vi "Tektronix AFG 3000 Series Generate Arbitrary Waveform Pulse.vi"() -> ()   [LabVIEW 2019]
doc: "Demonstrates how to configure then create an arbitrary waveform."
uses:
  <userlib>/Tektronix AFG 3000 Series/Tektronix AFG 3000 Series.lvlib
panel:
  out "Delta(ms)":u32
  out "taille(s)":i32
  out "periode(us)":dbl
  in  "LowLevel(V)":dbl
  in  "HighLevel(V)":dbl=1.0
  in  "Rise time(us)":dbl=1.0
  in  "Tau2 lenght(us)":dbl=1.0
  in  "Tau1 lenght(us)":dbl=1.0
  in  "Middle pulse lenght(us)":dbl=1.0
  in  "Init pulse lenght(us)":dbl=1.0
  out "Arbitrary Waveform Data":dbl[](array[numeric])
  out "Frequency (1000 Hz)":dbl=1000.0
  in  "DC Offset (0 V)":dbl
  in  "Gain (1 V)":dbl=1.0
  in  "Arbitrary Waveform Name (0: USER1)":u16(ring) items=["USER1", "USER2", "USER3", "USER4"]
  in  "Channel (0: Channel 1)":u16(ring) items=["Channel 1", "Channel 2"]
  in  "VISA resource name":refnum<visa-resource-name>
  # "(c) 2006-2012 National Instruments.  ALL RIGHTS RESERVED."
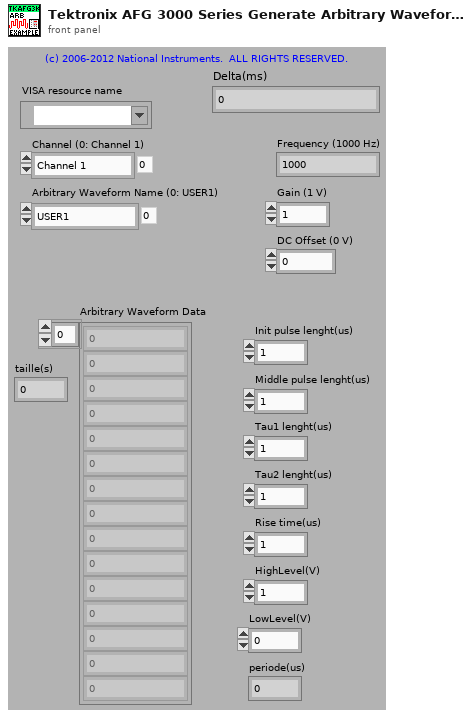
[diagram p1: front panel]
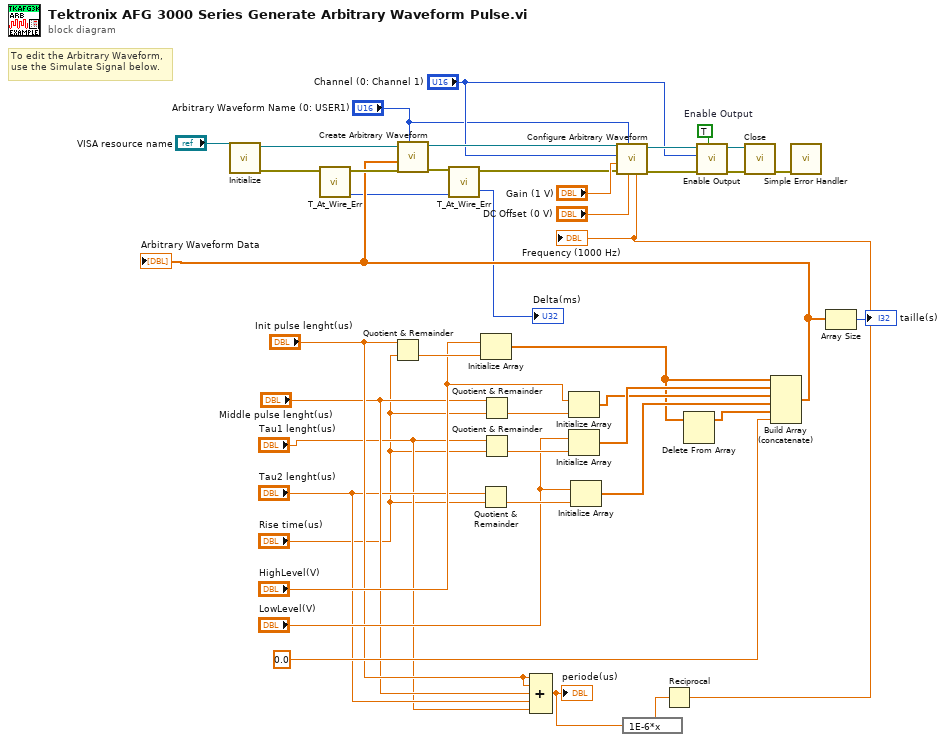
[diagram p0: block diagram]
diagram:
  w35 = TRUE  # Enable Output
  # "To edit the Arbitrary Waveform, use the Simulate Signal below."
  n1 = call <userlib>:"Initialize.vi"("VISA resource name"="VISA resource name") -> ("error out"=w9:errorcluster, "VISA resource name out"=w34:refnum<visa-resource-name>)  [unwired: 9 in]
  n2 = call <userlib>:"T_At_Wire_Err.vi"("error in (no error)"=w9) -> ("Clock(ms)"=w2:u32, "error out"=w8:errorcluster)  [unwired: 8 in, 1 out]
  n3 = Quotient & Remainder(x="Init pulse lenght(us)", y="Rise time(us)") -> (floor(x/y)=w29:dbl)  [unwired: 1 out]
  n4 = Initialize Array("HighLevel(V)", w29) -> (w16:dbl[])
  n5 = Quotient & Remainder(x="Tau2 lenght(us)", y="Rise time(us)") -> (floor(x/y)=w25:dbl)  [unwired: 1 out]
  n6 = Quotient & Remainder(x="Middle pulse lenght(us)", y="Rise time(us)") -> (floor(x/y)=w28:dbl)  [unwired: 1 out]
  n7 = Quotient & Remainder(x="Tau1 lenght(us)", y="Rise time(us)") -> (floor(x/y)=w26:dbl)  [unwired: 1 out]
  n8 = Compound Arithmetic op=ADD("Init pulse lenght(us)", "Init pulse lenght(us)", "Middle pulse lenght(us)", "Tau2 lenght(us)", "Tau1 lenght(us)") -> (w13:dbl)
  "periode(us)" <- w13
  n9 = Initialize Array("HighLevel(V)", w28) -> (w22:dbl[])
  n10 = Initialize Array("LowLevel(V)", w26) -> (w23:dbl[])
  n11 = Initialize Array("LowLevel(V)", w25) -> (w21:dbl[])
  n12 = expression code="1E-6*x"(w13) -> (w10:dbl)
  n13 = Reciprocal(x=w10) -> (1/x=w12:dbl)
  "Frequency (1000 Hz)" <- w12
  n14 = Delete From Array(array=w16) -> (array with subset deleted=w15:dbl[])  [unwired: 2 in, 1 out]
  n15 = Build Array (concatenate)(w16, w23, w22, w21, w15, 0.0) -> (w6:dbl[])
  "Arbitrary Waveform Data" <- w6
  n16 = call <userlib>:"Create Arbitrary Waveform.vi"("Arbitrary Waveform Name (0: USER1)"="Arbitrary Waveform Name (0: USER1)", "error in (no error)"=w8, "Arbitrary Waveform Data"=w6, "VISA resource name"=w34) -> ("error out"=w4:errorcluster, "VISA resource name out"=w37:refnum<visa-resource-name>)  [unwired: 6 in]
  n17 = call <userlib>:"T_At_Wire_Err.vi"("InitClock(ms)"=w2, "error in (no error)"=w4) -> ("error out"=w3:errorcluster, "Delta(ms)"=→"Delta(ms)":u32)  [unwired: 7 in, 1 out]
  n18 = call <userlib>:"Configure Arbitrary Waveform.vi"("Frequency (1000 Hz)"=w12, "DC Offset (0 V)"="DC Offset (0 V)", "Arbitrary Waveform Name (0: USER1)"="Arbitrary Waveform Name (0: USER1)", "error in (no error)"=w3, "Gain (1 V)"="Gain (1 V)", "Channel (0: Channel 1)"="Channel (0: Channel 1)", "VISA resource name"=w37) -> ("error out"=w7:errorcluster, "VISA resource name out"=w38:refnum<visa-resource-name>)  [unwired: 3 in]
  n19 = call <userlib>:"Enable Output.vi"("Enable Output (T: Enable)"=w35, "error in (no error)"=w7, "Channel (0: Channel 1)"="Channel (0: Channel 1)", "VISA resource name"=w38) -> ("error out"=w39:errorcluster, "VISA resource name out"=w40:refnum<visa-resource-name>)  [unwired: 5 in]
  n20 = call <userlib>:"Close.vi"("error in (no error)"=w39, "VISA resource name"=w40) -> ("error out"=w41:errorcluster)  [unwired: 9 in]
  n21 = call <vilib>:"Simple Error Handler.vi"("error in (no error)"=w41) -> ()  [unwired: 4 in, 5 out]
  n22 = Array Size(array=w6) -> (size(s)=→"taille(s)":i32)
